vi "block.vi"(2 "white":bool[][](array[boolean]), 4 "black":bool[][](array[boolean])) -> (1 "forbidden":bool[][](array[boolean]))   [LabVIEW 2014]
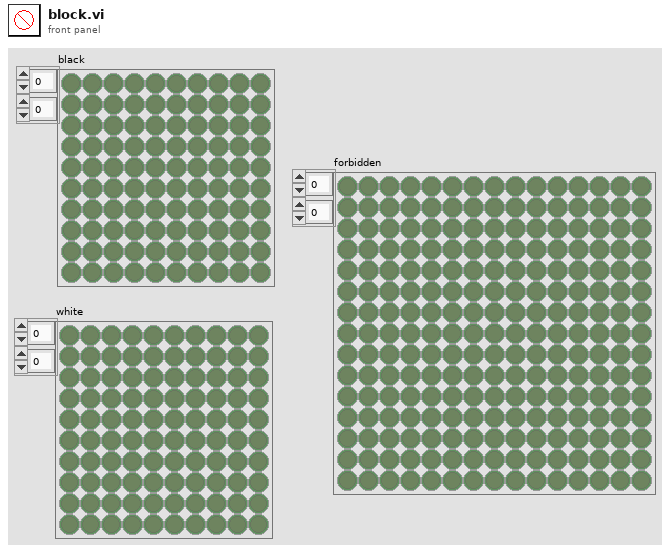
[diagram p1: front panel]
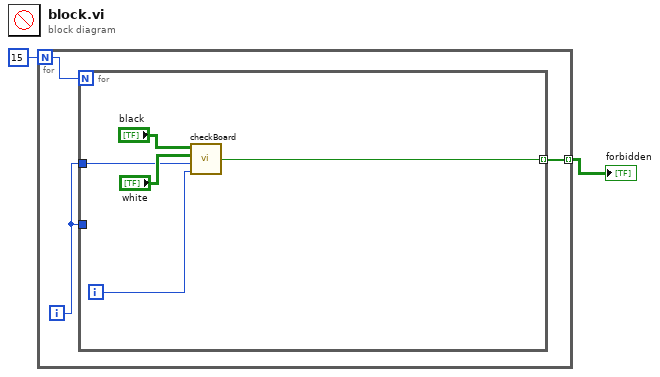
[diagram p0: block diagram]
diagram:
  n1 = for {
    N: 15 -> [w5]
    tunnel: [w3] -> w1 mode=indexing
    i -> [w4]
    n2 = for {
      N: w5 -> [_]
      tunnel: w4 -> [w9]
      tunnel: w4 -> [_]
      tunnel: [w6] -> w3 mode=indexing
      i -> [w8]
      n3 = call "checkBoard.vi"("column"=w8, "row"=w9, "white"="white", "black"="black") -> ("element"=w6:bool)
    }
  }
  "forbidden" <- w1
